vi "RunTimeButtonUI.vi"() -> ()   [LabVIEW 2019, in "RunTimeButton.lvclass"]
uses:
  RunTimeButton.lvclass
  <vilib>/NI/Configuration Framework/Node/NodeRef.ctl
  <vilib>/NI/Configuration Framework/Node/NISE_CEF_Node.lvclass
  <vilib>/NI/AMC/Message Queue.ctl
  <vilib>/NI/AMC/Message.ctl
  <vilib>/NI/Tools/Keyed Array/KeyedArray.ctl
  <vilib>/NI/Configuration Framework/Node/UserEventRef.ctl
  <vilib>/NI/Configuration Framework/Controls/EventCluster.ctl
  System.Windows.Forms
  C:/Program Files (x86)/National Instruments/LabVIEW 2019/vi.lib/NI/Configuration Framework/Node/NISE_CEF_Node.lvclass
  RunTimeButton.lvclass/RunTimeButton.ctl
  Read Button Properties.vi
  Write Button Properties.vi
  <vilib>/NI/AMC/Create Single Message.vi
  <vilib>/NI/AMC/Update Message Routing Info.vi
  <vilib>/NI/AMC/Send Message.vi
  <vilib>/NI/AMC/AMC.lvlib
  Configuration Tool.lvlib
  <vilib>/NI/Tools/Keyed Array/Tools_KeyedArray.lvlib
  <vilib>/NI/Configuration Framework/NISE_CEF_TreeControl.lvlib
panel:
  in  "Main UI Tab":T1(tab)
  in  "ID":string
  in  "Referenced GUID":string="9b525fa0-4d4a-4ec1-902b-bfeef88ebbcc"
  in  "Button Type":T2(ring)
  in  "Button Text":string
  in  "Caption":string
  in  "Tip Strip":string
  in  "Documentation":string
  in  "Glyph":refnum<k24>(container)
  in  "Host Path to Glyph":path
  in  "Host Path to Dependency File":path
  in  "Dependency Behavior":enum16{"Static", "Dynamic"}(ring)
  in  "user event":T3
  in  "main queue":T4
  in  "node ref":T5
  # "Display Settings"
  # "Action Settings"
  # "Dependency Settings"
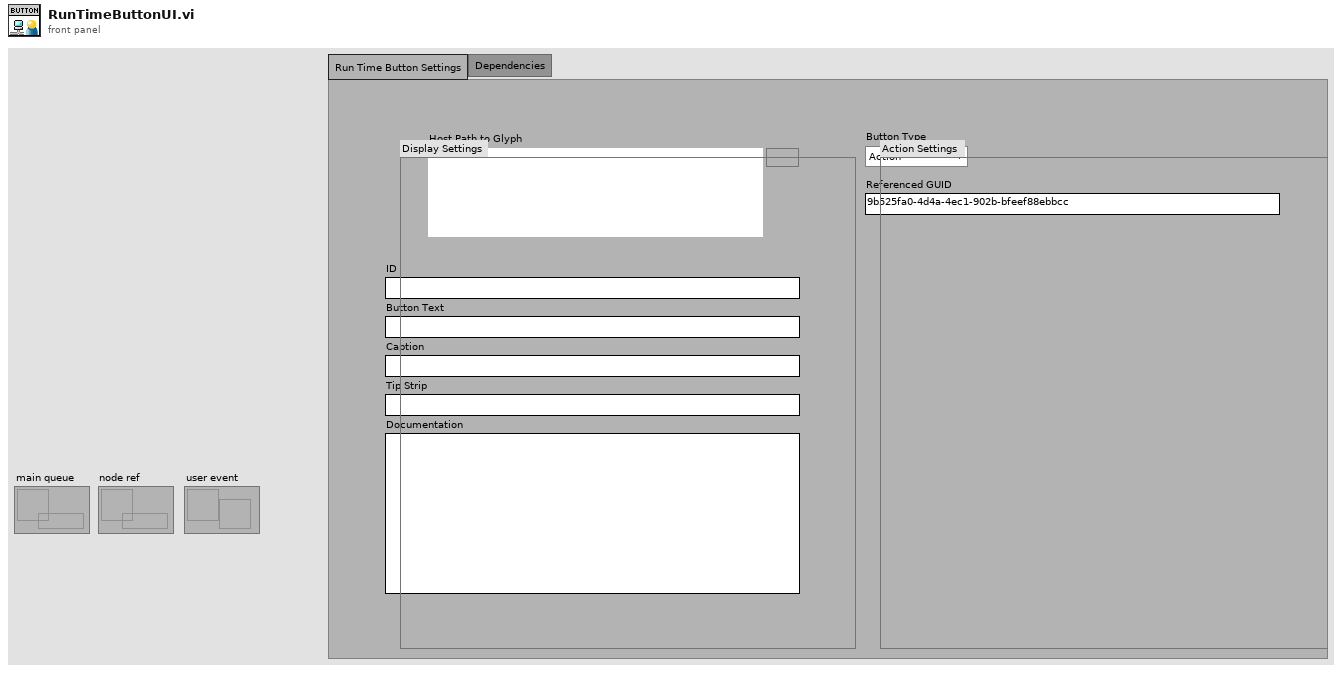
[diagram p1: front panel]
types:
  T1 = enum32{"Run Time Button Settings", "Dependencies"}
  T2 = enum16{"Action", "Dialog", "Page", "Notification", "Separator"}
  T3 = typedef "NISE_CEF_Node.lvclass/UserEventRef.ctl" = refnum<user-event>
  T4 = typedef "AMC.lvlib/Message Queue.ctl" = refnum<queue>
  T5 = typedef "NISE_CEF_Node.lvclass/NodeRef.ctl" = refnum<data-value>
  T6 = typedef "VeriStand Custom Device XML Parser.lvlib/ButtonLists Properties.ctl" = cluster{"ID":string, "Glyph":T7, "Button Type":T8, "Referenced GUID":string, "Button Text":string, "Caption":string, "Tip Strip":string, "Documentation":string, "Dependency":T9}
  T7 = typedef "VeriStand Custom Device XML Parser.lvlib/Path Cluster.ctl" = cluster{"Path":path, "Path Type":enum16{"Absolute", "To Base", "To Common Doc Dir", "To Application Data Dir"}}
  T8 = typedef "VeriStand Custom Device XML Parser.lvlib/Button Type.ctl" = enum16{"Action", "Dialog", "Page", "Notification", "Separator"}
  T9 = typedef "VeriStand Custom Device XML Parser.lvlib/Dependency Properties.ctl" = cluster{"File Path Control":path, "Path Type":enum16{"Absolute", "To Base", "To Common Doc Dir", "To Application Data Dir"}, "Behavior":enum16{"Static", "Dynamic"}}
  T10 = enum16{"Absolute", "To Base", "To Common Doc Dir", "To Application Data Dir"}
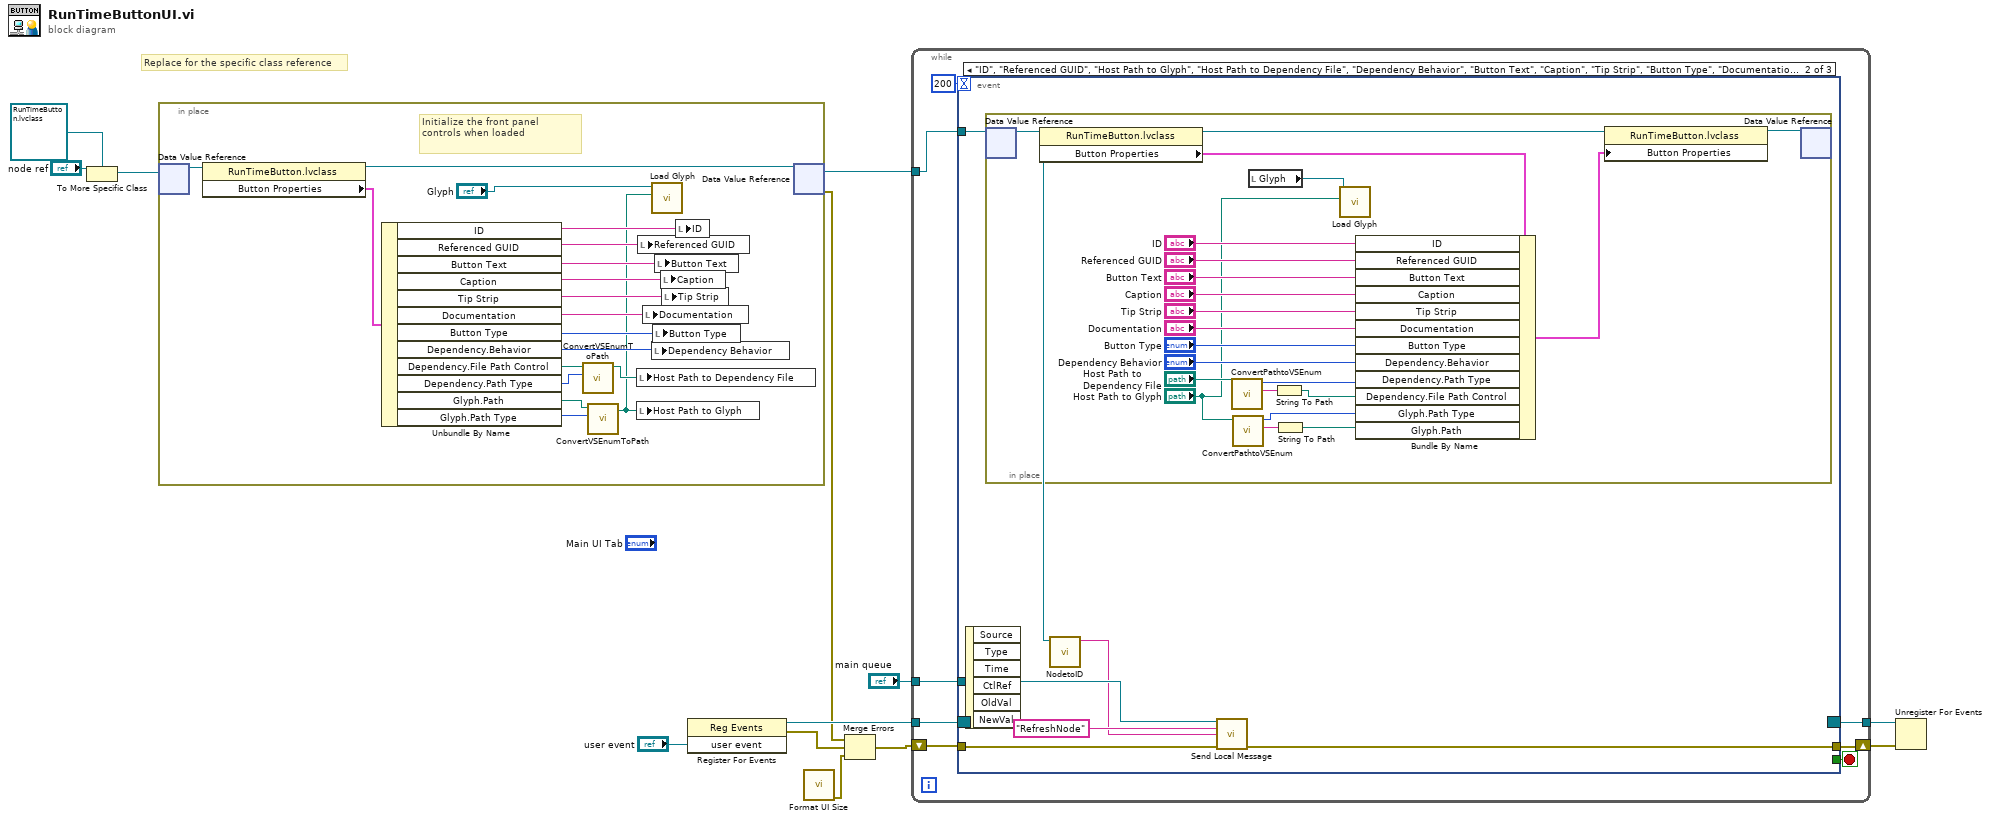
[diagram p0: block diagram]
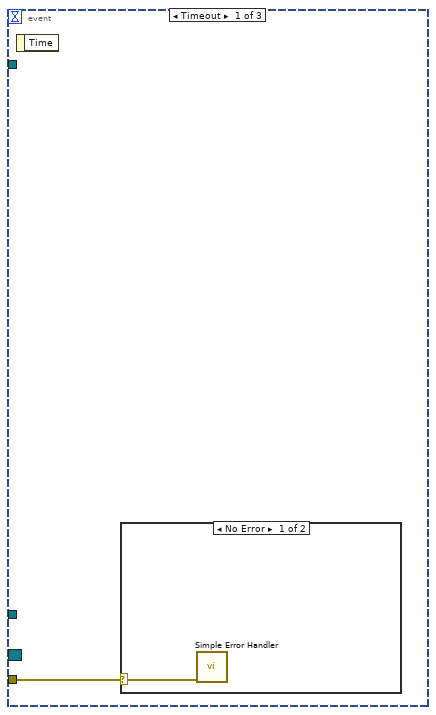
[diagram p2: hidden frame]
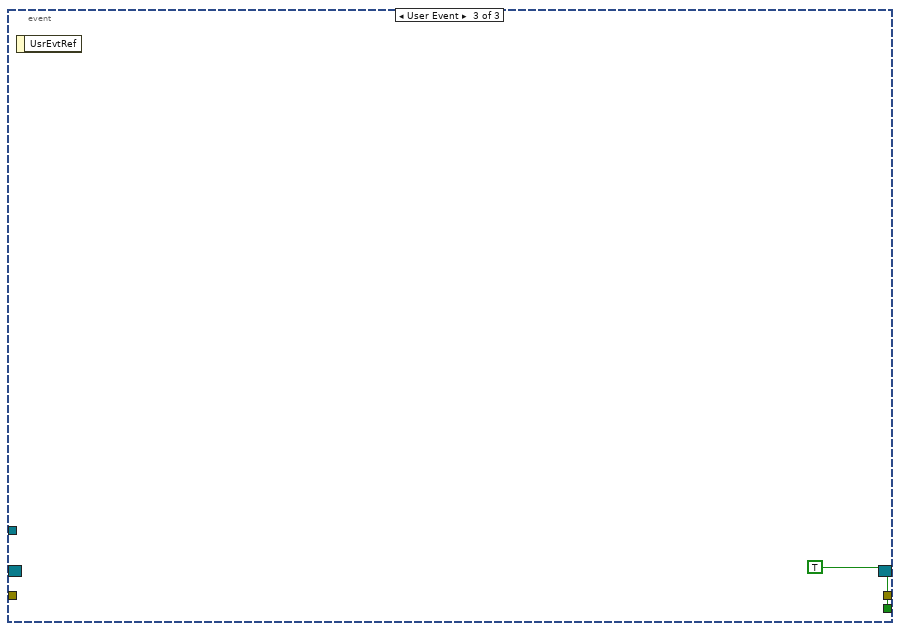
[diagram p4: hidden frame]
diagram:
  # "Replace for the specific class reference"
  n1 = To More Specific Class(target class=refnum<data-value> refnum ("data value reference"), reference="node ref") -> (specific class reference=w6:refnum<data-value>)  [unwired: 1 in, 1 out]
  n2 = in-place {
    # "Initialize the front panel controls when loaded"
    n3 = in-place-dvr #1(w6) -> (w31:refnum<class "RunTimeButton.lvclass">)  [unwired: 1 out]
    n4 = property class="RunTimeButton.lvclass"(reference=w31) -> (reference out=w30:refnum<class "RunTimeButton.lvclass">, "Button Properties"=w29:T6)  [unwired: 1 in, 1 out]
    n5 = Unbundle By Name(w29) -> ("ID"=w28:string, "Referenced GUID"=w27:string, "Button Text"=w26:string, "Caption"=w25:string, "Tip Strip"=w24:string, "Documentation"=w23:string, "Button Type"=w22:T8, "Dependency.Behavior"=w21:enum16{"Static", "Dynamic"}, "Dependency.File Path Control"=w20:path, "Dependency.Path Type"=w19:T10, "Glyph.Path"=w17:path, "Glyph.Path Type"=w16:T10)
    n6 = call "ConvertVSEnumToPath.vi"("Source.Path Type"=w19, "Path In"=w20) -> ("appended path"=w18:path)  [unwired: 9 in]
    n7 = call "ConvertVSEnumToPath.vi"("Source.Path Type"=w16, "Path In"=w17) -> ("appended path"=w14:path)  [unwired: 9 in]
    n8 = local write "Host Path to Dependency File"(w18) -> ()
    n9 = local write "Host Path to Glyph"(w14) -> ()
    n10 = local write "Referenced GUID"(w27) -> ()
    n11 = local write "Documentation"(w23) -> ()
    n12 = call "Load Glyph.vi"("Path"=w14, "PictureBox in"="Glyph") -> ()  [unwired: 8 in, 2 out]
    n13 = local write "Dependency Behavior"(w21) -> ()
    n14 = local write "Button Type"(w22) -> ()
    n15 = local write "Button Text"(w26) -> ()
    n16 = local write "Caption"(w25) -> ()
    n17 = local write "Tip Strip"(w24) -> ()
    n18 = local write "ID"(w28) -> ()
    n19 = in-place-dvr #1(w30) -> (w13:refnum<data-value>, w3:errorcluster)
  }
  n20 = register-events("user event") -> (reference out=w10:refnum<event-registration>, error out=w4:errorcluster)  [unwired: 2 in]
  n21 = call "Format UI Size.vi"() -> ("error out"=w1:errorcluster)  [unwired: 11 in]
  n22 = Merge Errors(w3, w4, w1) -> (w2:errorcluster)
  n23 = while {
    tunnel: w13 -> [w39]
    tunnel: "main queue" -> [w38]
    tunnel: w10 -> [w36]
    tunnel: [w35] -> w9
    shift-right: [w33] -> w8
    shift-left: w2 -> [w32]
    stop <- w34 stop-if-true
    n24 = event shown="[1] \"ID\", \"Referenced GUID\", \"Host Path to Glyph\", \"Host Path to Dependency File\", \"Dependency Behavior\", \"Button Text\", \"Caption\", \"Tip Strip\", \"Button Type\", \"Documentation\": Value Change" {
      selector: w36 -> [_ _ _]
      dyn-events: [_ _ _] -> w35
      timeout: 200 -> [_ _ _]
      tunnel: w39 -> [_ w45 _]
      tunnel: w38 -> [_ w46 _]
      tunnel: [_ _ TRUE] -> w34
      tunnel: [_ w43 _] -> w33
      tunnel: w32 -> [w40 w42 _]
      event Timeout {
        n25 = event-data() -> ()  [unwired: 1 in, 1 out]
        n26 = case shown="No Error" w40 {
          selector: w40 -> [w41 _]
          frame No Error {
            n27 = call <vilib>:"Simple Error Handler.vi"("error in (no error)"=w41) -> ()  [unwired: 4 in, 5 out]
          }
          frame Error {
          }
        }
      }
      event "ID", "Referenced GUID", "Host Path to Glyph", "Host Path to Dependency File", "Dependency Behavior", "Button Text", "Caption", "Tip Strip", "Button Type", "Documentation": Value Change {
        n28 = event-data() -> ()  [unwired: 1 in, 6 out]
        n29 = in-place {
          n30 = in-place-dvr #2(w45) -> (w67:refnum<class "RunTimeButton.lvclass">)  [unwired: 1 out]
          n31 = property class="RunTimeButton.lvclass"(reference=w67) -> (reference out=w66:refnum<class "RunTimeButton.lvclass">, "Button Properties"=w65:T6)  [unwired: 1 in, 1 out]
          n32 = call "ConvertPathtoVSEnum.vi"("Path In"="Host Path to Dependency File") -> ("Remaining Path"=w68:string, "VS Enum Out"=w54:T10)  [unwired: 9 in]
          n33 = call "ConvertPathtoVSEnum.vi"("Path In"="Host Path to Glyph") -> ("Remaining Path"=w52:string, "VS Enum Out"=w50:T10)  [unwired: 9 in]
          n34 = local read "Glyph"() -> (w49:refnum<k24>)
          n35 = String To Path(string=w68) -> (path=w53:path)
          n36 = String To Path(string=w52) -> (path=w51:path)
          n37 = call "Load Glyph.vi"("Path"="Host Path to Glyph", "PictureBox in"=w49) -> ()  [unwired: 8 in, 2 out]
          n38 = Bundle By Name(cluster=w65, "ID"="ID", "Referenced GUID"="Referenced GUID", "Button Text"="Button Text", "Caption"="Caption", "Tip Strip"="Tip Strip", "Documentation"="Documentation", "Button Type"="Button Type", "Dependency.Behavior"="Dependency Behavior", "Dependency.Path Type"=w54, "Dependency.File Path Control"=w53, "Glyph.Path Type"=w50, "Glyph.Path"=w51) -> (w64:T6)
          n39 = property class="RunTimeButton.lvclass"(reference=w66, "Button Properties"=w64) -> (reference out=w69:refnum<class "RunTimeButton.lvclass">)  [unwired: 1 in, 1 out]
          n40 = in-place-dvr #2(w69) -> ()  [unwired: 2 out]
        }
        n41 = call <vilib>:"NodetoID.vi"("node ref"=w45) -> ("ID"=w44:string)  [unwired: 9 in, 1 out]
        n42 = call <vilib>:"Send Local Message.vi"("message queue in"=w46, "message name"="RefreshNode" ("Message Name"), "message value"=w44, "error in"=w42) -> ("error out"=w43:errorcluster)  [unwired: 9 in, 2 out]
      }
      event User Event {
        n43 = event-data() -> ()  [unwired: 1 in, 1 out]
      }
    }
  }
  n44 = Unregister For Events(event registration refnum=w9, error in=w8) -> ()  [unwired: 1 out]
